vi "hidSPD Open Session.vi"(8 "error in (no error)":errorcluster, 11 "HidDevInfo":T2) -> (0 "error out":errorcluster, 3 "spdDevSession out":T1)   [LabVIEW 2018, in "hidSPDLibForLabView.lvlib"]
uses:
  hidSPDLibForLabView.lvlib
  hidSPD Controls/hidSPD HidDevInfo.ctl
  hidSPD Controls/hidSPD Device Session.ctl
  <vilib>/Utility/error.llb/Error Cluster From Error Code.vi
  <vilib>/ErrorRing/Error Ring.xnode
  hidSPD DLL files/libSPD.dll
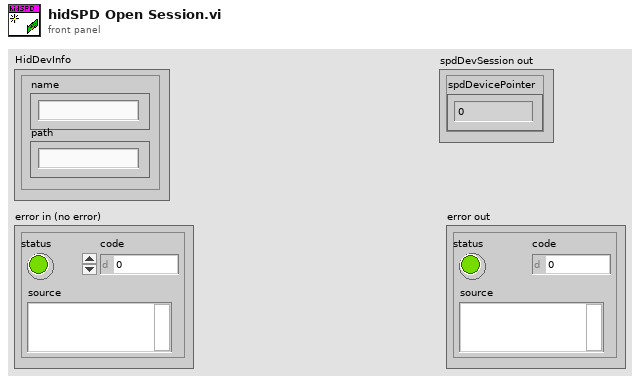
[diagram p1: front panel]
types:
  T1 = typedef "hidSPDLibForLabView.lvlib/hidSPD Device Session.ctl" = cluster{"spdDevicePointer":u64}
  T2 = typedef "hidSPDLibForLabView.lvlib/hidSPD HidDevInfo.ctl" = cluster{"name":string, "path":string}
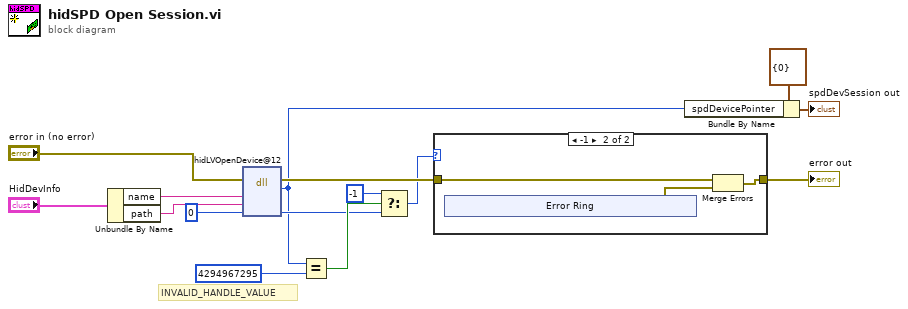
[diagram p0: block diagram]
diagram:
  # "INVALID_HANDLE_VALUE"
  n1 = Unbundle By Name("HidDevInfo") -> ("name"=w10:string, "path"=w9:string)
  n2 = dll-call lib="D:/NextCloud/SPD/hidSPDLibForLabView/hidSPD DLL files/libSPD.dll" fn="hidLVOpenDevice@12"(error in="error in (no error)", "deviceName"=w10, "devicePath"=w9, "errorCode"=0 ("deguflength")) -> (error out=w14:errorcluster, "spdDevHandle"=w2:u64, "errorCode"=w6:i32)  [unwired: 4 in, 1 out]
  n3 = Equal?(x=w2, y=u64 4294967295) -> (x = y?=w7:bool)
  n4 = Select(t=-1, s=w7, f=w6) -> (s? t:f=w4:i32)
  n5 = case shown="-1" w4 {
    tunnel: w14 -> [w16 w19]
    tunnel: [w16 w17] -> w13
    frame 0, Default {
    }
    frame -1 {
      n6 = xnode "Error Ring"() -> ("error out"=w18:errorcluster)
      n7 = Merge Errors(w19, w18) -> (w17:errorcluster)
    }
  }
  "error out" <- w13
  n8 = Bundle By Name(cluster=T1 {"spdDevicePointer"=0} ("spdDeviceSession"), "spdDevicePointer"=w2) -> (→"spdDevSession out":T1)
